vi "_fgv_range_tables.vi"(5 "Numeric Value in (0.0)":dbl, 6 "Range Tables (empty)":T2[](array[typedef]) {"Type" items=["Range", "Coerced", "Discrete"]}, 7 "Operation":T3=enum."Check", 8 "error in":errorcluster caption="error in (no error)", 9 "String value in (\"\")":string, 10 "Range Table ID in":string, 11 "VISA resource name":refnum<visa-resource-name>) -> (0 "error out":errorcluster, 1 "String Value out":string, 2 "Range Table Type out":T1, 3 "VISA resource name out":refnum<visa-resource-name>, 4 "Numeric Value out":dbl)   [LabVIEW 2020, in "Rohde&Schwarz RTx Oscilloscopes.lvlib" / "rsidr_core.lvlib"]
uses:
  rsidr_core.lvlib
  _type_Operation_Fgv_RangeTable.ctl
  type_Input_Format_RangeTable.ctl
  _type_RangeTable_Type.ctl
  type_Error_Codes.ctl
  type_AdditionalFlag_Bits.ctl
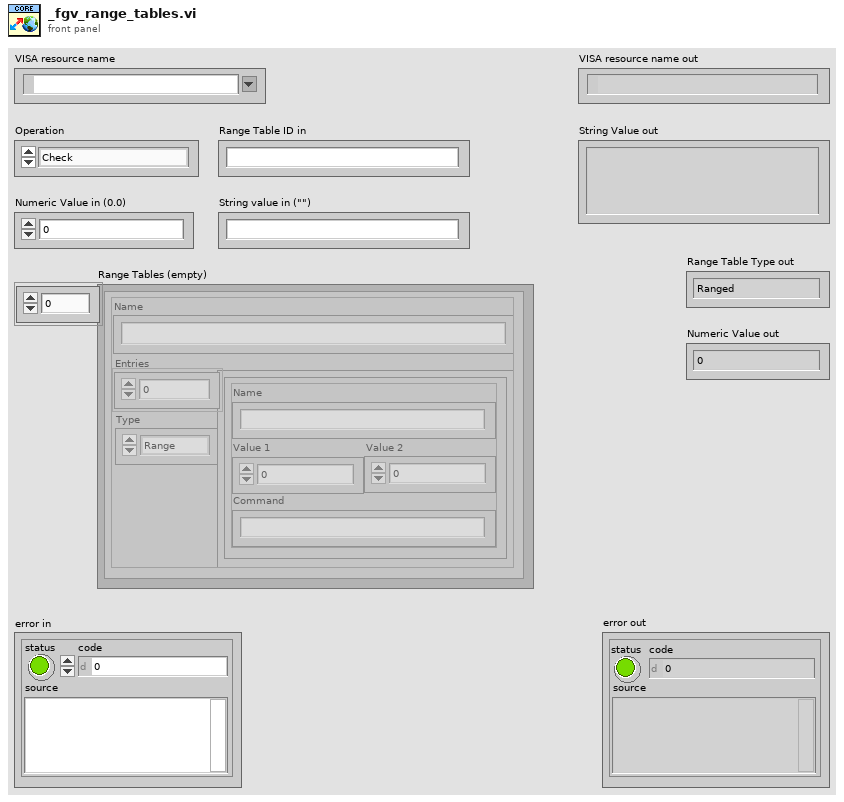
[diagram p1: front panel]
types:
  T1 = typedef "Rohde&Schwarz RTx Oscilloscopes.lvlib/rsidr_core.lvlib/_type_RangeTable_Type.ctl" = enum16{"Ranged", "Coerced", "Discrete"}
  T2 = typedef "Rohde&Schwarz RTx Oscilloscopes.lvlib/rsidr_core.lvlib/type_Input_Format_RangeTable.ctl" = cluster{"Type":u16, "Name":string, "Entries":cluster{"Name":string, "Value 1":dbl, "Value 2":dbl, "Command":string}[]}
  T3 = typedef "Rohde&Schwarz RTx Oscilloscopes.lvlib/rsidr_core.lvlib/_type_Operation_Fgv_RangeTable.ctl" = enum16{"Initialize", "Check", "Coerce", "Get Command String", "Get Numeric Value", "Get Default Value", "Get Range Table Type"}
  T4 = typedef "Rohde&Schwarz RTx Oscilloscopes.lvlib/rsidr_core.lvlib/type_Error_Codes.ctl" = enum16{"No_error", "VISA_err_ResourceNotFound", "VISA_err_Timeout", "VISA_warn_MoreDataAvailable", "RS_err_MissingCallback", "RS_err_InvalidAttribute", "RS_err_InvalidValue", "RS_err_UnknownResource", "RS_err_AlreadyInitialized", "RS_err_InstrumentStatus", "RS_err_BadRepCapName", "RS_err_TypesMismatch", "RS_err_ValueNotSupported", "RS_err_InvalidRngTable", "RS_err_IDqueryFail", "RS_err_UnexpResponse", "VISA_warn_ConfigNotLoaded", "RS_err_AttributeNotReadable", "RS_err_AttributeNotWritable", "RS_err_InstrumentType", "RS_err_InstrumentOption", "VISA_err_InvalidSize", "RS_err_ReliabilityIndicator", "VISA_warn_UnknownStatus", "VISA_warn_TermCharRead", "VISA_err_IO_error", "RS_err_FunctionNotSupported", "VISA_warn_QueueEmpty"}
  T5 = typedef "Rohde&Schwarz RTx Oscilloscopes.lvlib/rsidr_core.lvlib/type_AdditionalFlag_Bits.ctl" = enum16{"Send LF after Bin Block", "Junk read with io_clear_buffers.vi", "io_clear_buffers: viClear()", "io_clear_buffers: viFlush()", "<NotUsed1>", "Allow Dbl & Int Bin/Ascii read", "*OPC? in check_instrument_error.vi", "<NotUsed2>", "Smart Enum Matching", "Less Strict RepCaps check", "AssureResponseEndWithLF"}
  T6 = cluster{"Values":i32[], "FullCmd":string[], "ShortCmd":string[]}
  T7 = cluster{"Name":string, "Value 1":dbl, "Value 2":dbl, "Command":string}[]
  T8 = cluster{"Name":string, "Value 1":dbl, "Value 2":dbl, "Command":string}
  T9 = cluster{"Name":string, "Range Table Type":T1, "Variant":variant}
  T10 = cluster{"Name":string, "Range Table Type":T1, "Variant":variant}[]
  T11 = typedef "Rohde&Schwarz RTx Oscilloscopes.lvlib/rsidr_core.lvlib/type_Session_Data.ctl" = cluster{"IDN string":string, "Instrument FW":string, "Instr type":string, "Instr type for err. msg.":string, "Installed Options":string[], "Ignore Error Messages":string, "Logging params":variant, "OPC Timeout":i32, "VISA Timeout":i32, "STB Poll VISA Timeout":i32, "Additional Flags":i32, "Wait Before Read":i32, "Wait Before Write":i32, "Option String Flags":i32, "IO Segment Size":i64, "VISA Access Mode":T12, "Interface Type":T13, "OPC Wait Mode":T14, "Bin Float Number  Format":T15, "Bin Integer Number Format":T16, "Simulate":bool, "VXIcapable":bool, "Duplicate Session":bool, "Add LF to Write":bool, "Logging":bool, "Fast Sweep":bool, "Query Instrument Status":bool, "Check Range":bool, "Check Options":bool, "OPC-sync Attr Writes":bool, "OPC-sync Attr Queries":bool}
  T12 = typedef "Rohde&Schwarz RTx Oscilloscopes.lvlib/rsidr_core.lvlib/type_VisaAccessMode.ctl" = u16
  T13 = typedef "Rohde&Schwarz RTx Oscilloscopes.lvlib/rsidr_core.lvlib/type_InterfaceType.ctl" = enum16{"Unknown", "GPIB", "VXI", "GPIB_VXI", "ASRL", "PXI", "TCPIP", "USB", "SOCKET"}
  T14 = typedef "Rohde&Schwarz RTx Oscilloscopes.lvlib/rsidr_core.lvlib/type_OPC_Wait_Mode.ctl" = enum16{"STBpolling", "STBpollingSlow", "STBpollingSuperSlow", "ServiceRequest", "OPCquery"}
  T15 = typedef "Rohde&Schwarz RTx Oscilloscopes.lvlib/rsidr_core.lvlib/type_Binary_Float_Number_Format.ctl" = enum16{"Float_4_Bytes_Swapped", "Float_4_Bytes", "Double_8_Bytes_Swapped", "Double_8_Bytes"}
  T16 = typedef "Rohde&Schwarz RTx Oscilloscopes.lvlib/rsidr_core.lvlib/type_Binary_Integer_Number_Format.ctl" = enum16{"Int32_4_Bytes_Swapped", "Int32_4 Bytes", "Int16_2_Bytes_Swapped", "Int16_2_Bytes"}
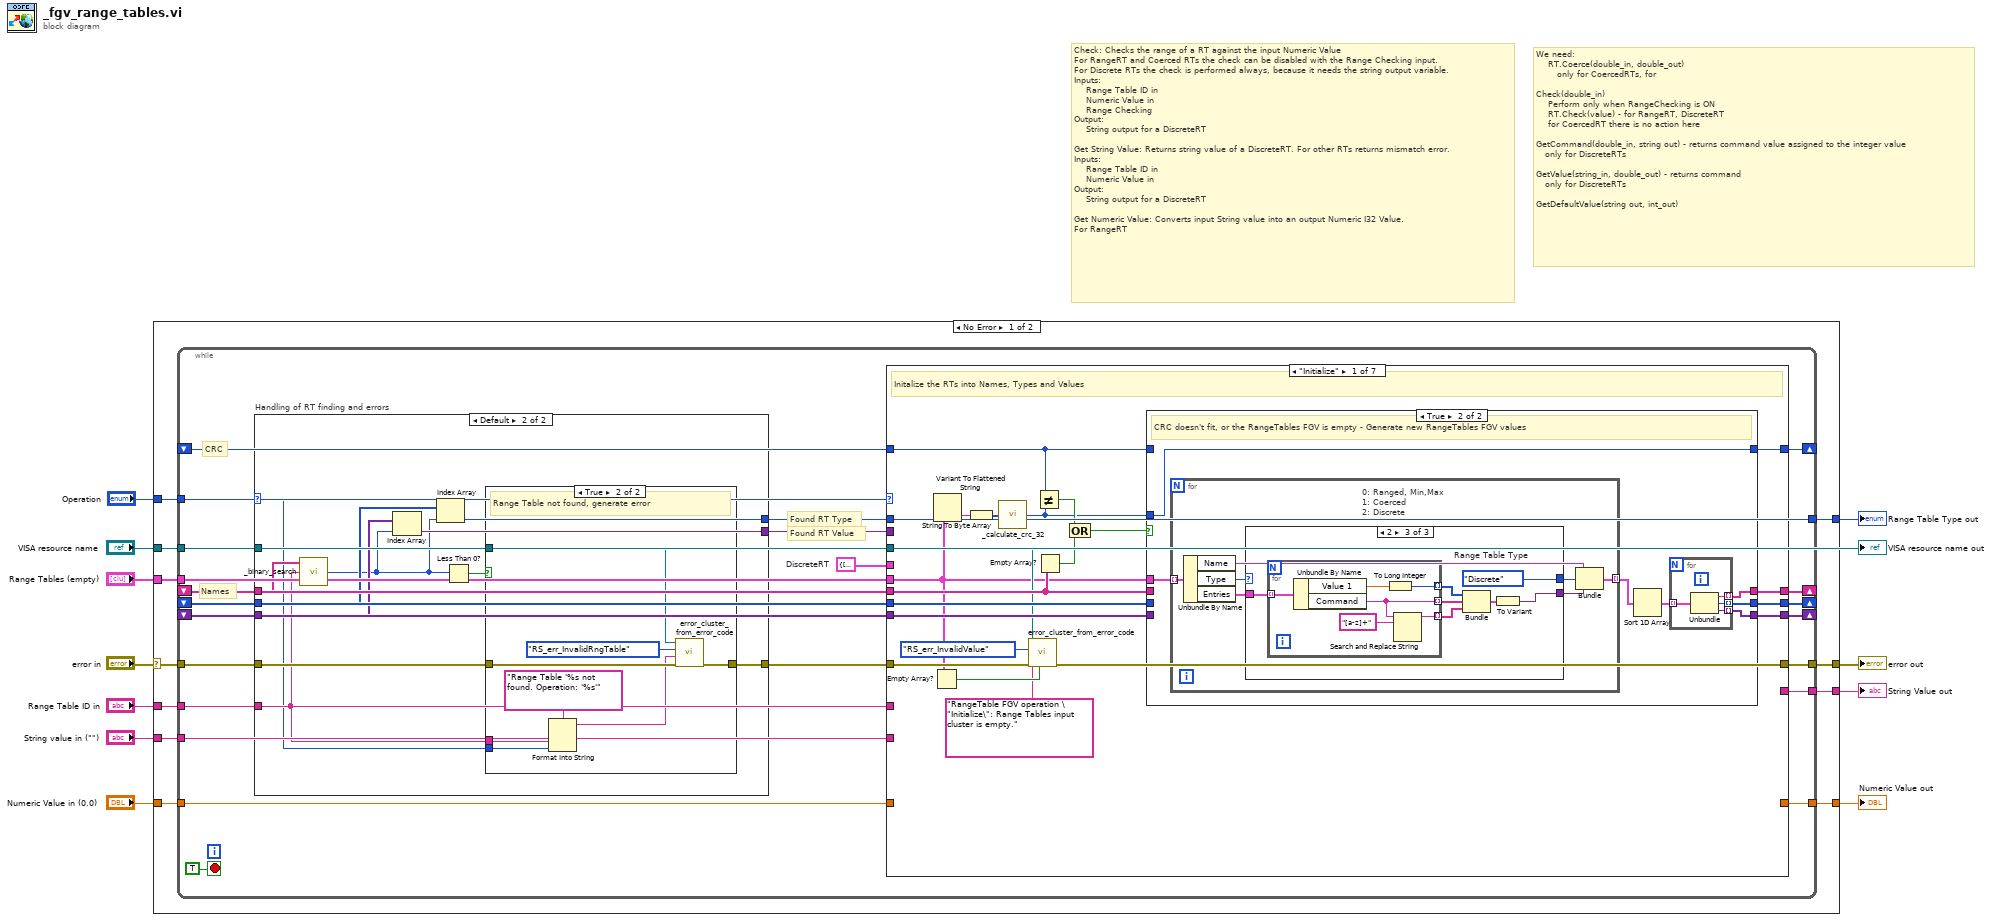
[diagram p0: block diagram]
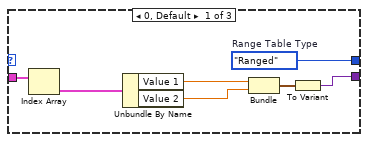
[diagram p5: hidden frame]
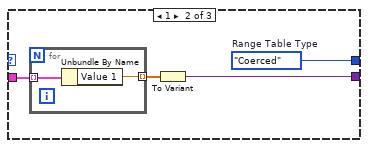
[diagram p6: hidden frame]
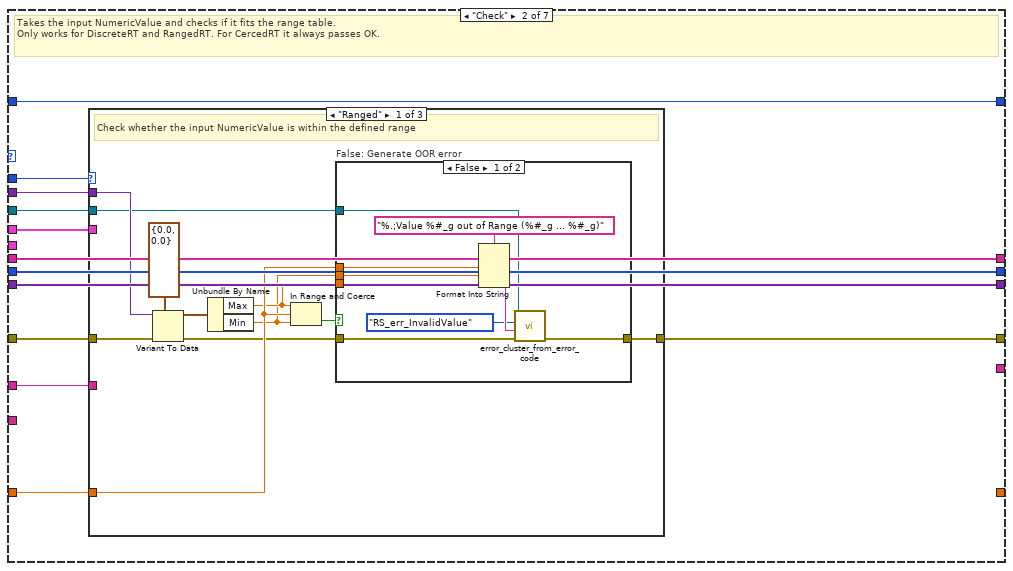
[diagram p7: hidden frame]
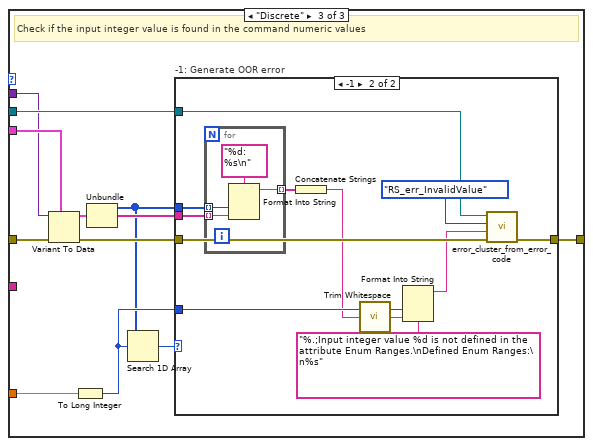
[diagram p10: hidden frame]
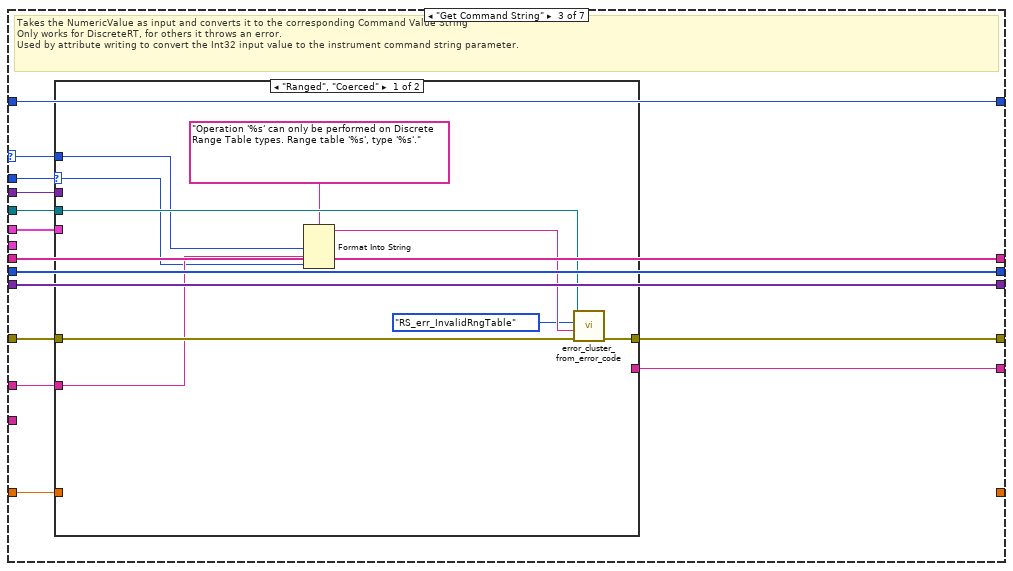
[diagram p12: hidden frame]
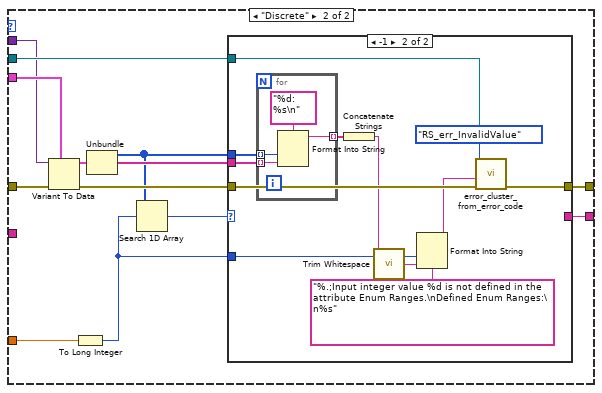
[diagram p13: hidden frame]
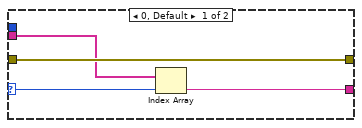
[diagram p14: hidden frame]
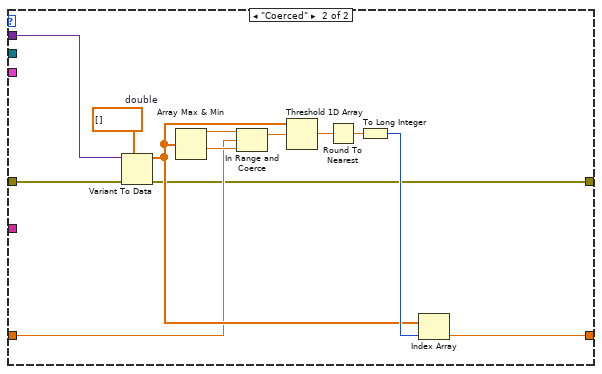
[diagram p16: hidden frame]
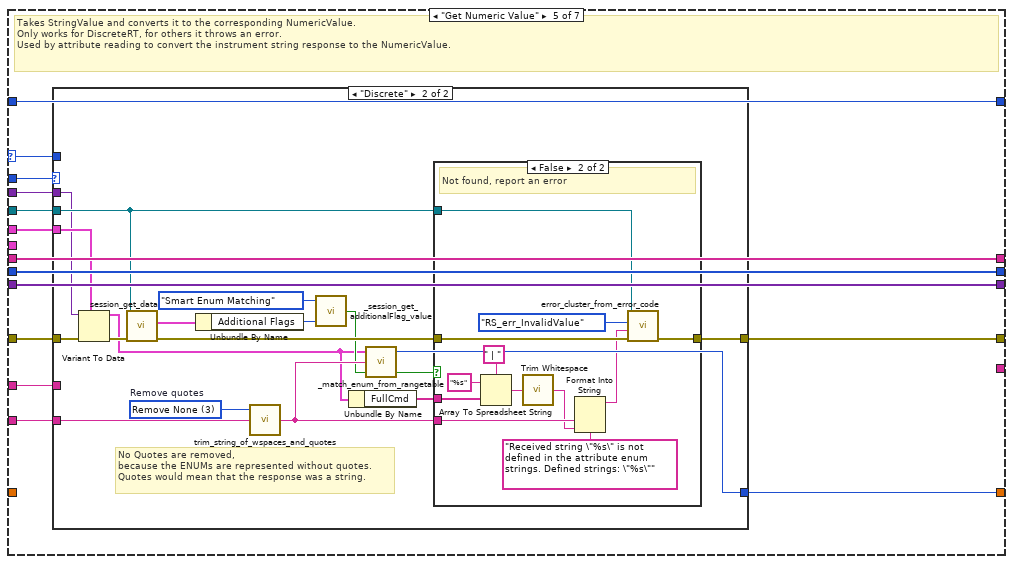
[diagram p17: hidden frame]
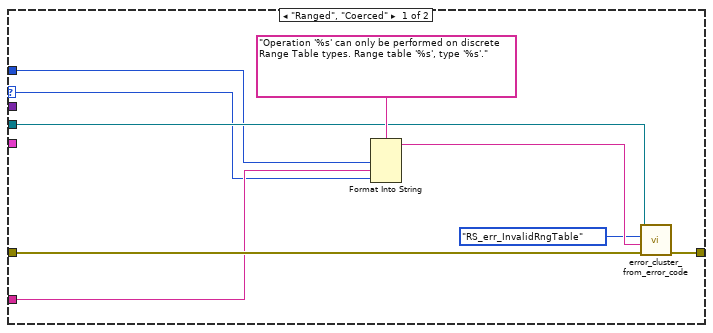
[diagram p18: hidden frame]
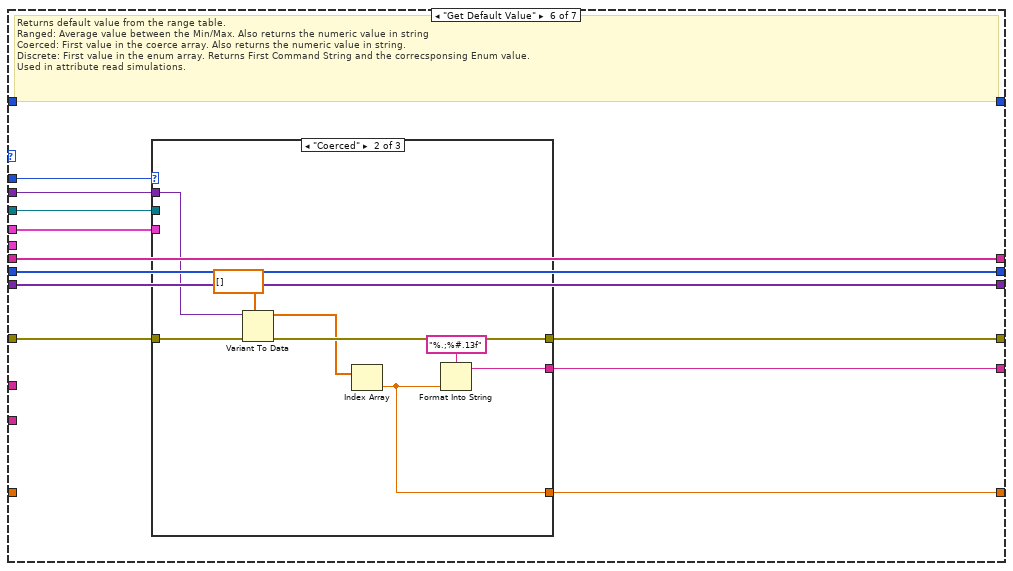
[diagram p20: hidden frame]
diagram:
  # "We need:\n    RT.Coerce(double_in, double_out)\n       only for CoercedRTs, for \n\nCheck(double_in)\n    Perform only when RangeChecking is ON\n    RT.Check(value) - for RangeRT, DiscreteRT\n    for CoercedRT there is no action here\n\nGetCommand(double_in, string out) - returns command value assigned to the integer value\n   only for DiscreteRTs\n\nGetValue(string_in, double_out) - returns command \n   only for DiscreteRTs\n\nGetDefaultValue(string out, int_out)"
  # "Check: Checks the range of a RT against the input Numeric Value\nFor RangeRT and Coerced RTs the check can be disabled with the Range Checking input.\nFor Discrete RTs the check is performed always, because it needs the string output variable.\nInputs:\n    Range Table ID in\n    Numeric Value in\n    Range Checking\nOutput:\n    String output for a DiscreteRT\n\nGet String Value: Returns string value of a DiscreteRT. For other RTs returns mismatch error.\nInputs:\n    Range Table ID in\n    Numeric Value in\nOutput:\n    String output for a DiscreteRT\n\nGet Numeric Value: Converts input String value into an output Numeric I32 Value.\nFor RangeRT"
  n1 = case shown="No Error" "error in" {
    selector: "error in" -> [w18 w384]
    tunnel: "Operation" -> [w22 _]
    tunnel: [w17 w384] -> w7
    tunnel: "Range Table ID in" -> [w21 _]
    tunnel: "Numeric Value in (0.0)" -> [w20 w383]
    tunnel: "String value in (\"\")" -> [w19 _]
    tunnel: [w16 _] -> w6
    tunnel: "VISA resource name" -> [w15 _]
    tunnel: "Range Tables (empty)" -> [w14 _]
    tunnel: [w13 w383] -> w2
    tunnel: [w12 _] -> w1
    frame No Error {
      n2 = while {
        tunnel: w22 -> [w32]
        tunnel: w21 -> [w34]
        tunnel: w20 -> [w45]
        tunnel: w19 -> [w44]
        tunnel: w18 -> [w31]
        tunnel: [w43] -> w17
        tunnel: [w42] -> w16
        shift-right: [w41] -> _
        shift-left: _ -> [w29]
        shift-right: [w39] -> _
        shift-left: _ -> [w27]
        shift-right: [w38] -> _
        shift-left: _ -> [w33]
        shift-right: [w36] -> _
        shift-left: _ -> [w37]
        tunnel: w15 -> [w28]
        tunnel: w14 -> [w35]
        tunnel: [w24] -> w13
        tunnel: [w23] -> w12
        stop <- TRUE stop-if-true
        w25 = T6 {"Values"=[], "FullCmd"=[], "ShortCmd"=[]}  # DiscreteRT
        # "Found RT Value"
        # "Found RT Type"
        # "CRC"
        # "Names"
        n3 = case "Handling of RT finding and errors" shown="Default" w32 {
          selector: w32 -> [_ w49]
          tunnel: w34 -> [_ w53]
          tunnel: w33 -> [_ w55]
          tunnel: w31 -> [w46 w57]
          tunnel: [w46 w58] -> w30
          tunnel: w29 -> [_ w54]
          tunnel: w28 -> [_ w56]
          tunnel: w27 -> [_ w52]
          tunnel: [_ w51] -> w26
          tunnel: [_ w50] -> w23
          frame "Initialize" {
          }
          frame Default {
            n4 = call "_binary_search.vi"("String to search"=w53, "Strings in"=w55) -> ("Index out"=w48:i32)  [unwired: 3 in]
            n5 = Index Array(array=w52, index=w48) -> (element=w51:variant)
            n6 = Index Array(array=w54, index=w48) -> (element=w50:T1)
            n7 = Less Than 0?(x=w48) -> (x < 0?=w47:bool)
            n8 = case shown="True" w47 {
              tunnel: [w59 w66] -> w58
              tunnel: w57 -> [w59 w65]
              tunnel: w56 -> [_ w64]
              tunnel: w53 -> [_ w63]
              tunnel: w49 -> [_ w60]
              frame False {
              }
              frame True {
                # "Range Table not found, generate error"
                n9 = Format Into String(format string="Range Table '%s not found. Operation: '%s'" ("string"), w63, w60) -> (resulting string=w62:string)  [unwired: 2 in, 1 out]
                n10 = call "error_cluster_from_error_code.vi"("error in"=w65, "Error Message (\"\")"=w62, "Error Enum in"=type_Error_Codes."RS_err_InvalidRngTable", "VISA resource name"=w64) -> ("error out"=w66:errorcluster)  [unwired: 6 in, 1 out]
              }
            }
          }
        }
        n11 = case shown="\"Initialize\"" w32 {
          selector: w32 -> [_ _ w200 w257 w286 _ _]
          tunnel: [w86 w148 w213 w269 w298 w349 w378] -> w43
          tunnel: w34 -> [_ w140 w204 w261 w295 _ _]
          tunnel: w44 -> [_ _ _ _ w297 _ _]
          tunnel: w45 -> [_ w147 w212 w268 _ _ _]
          tunnel: w30 -> [w85 w145 w209 w266 w294 w347 w378]
          tunnel: [_ _ w211 _ _ w342 _] -> w42
          tunnel: w29 -> [w80 w143 w207 w264 w293 w345 w379]
          tunnel: [w88 w143 w207 w264 w293 w345 w379] -> w41
          tunnel: w27 -> [w79 w144 w208 w265 w292 w346 w381]
          tunnel: [w87 w144 w208 w265 w292 w346 w381] -> w39
          tunnel: [w84 w146 w210 w267 w296 w348 w382] -> w38
          tunnel: w33 -> [w77 w146 w210 w267 w296 w348 w382]
          tunnel: w37 -> [w74 w142 w206 w263 w291 w344 w380]
          tunnel: [w73 w142 w206 w263 w291 w344 w380] -> w36
          tunnel: w28 -> [w69 w141 w205 w262 w290 w343 _]
          tunnel: w35 -> [w68 _ _ _ _ _ _]
          tunnel: w25 -> [_ w139 w203 w260 w289 w341 _]
          tunnel: w23 -> [_ w138 w201 w258 w287 w340 _]
          tunnel: w26 -> [_ w137 w202 w259 w288 w339 _]
          tunnel: [_ _ _ w256 w285 w338 _] -> w24
          frame "Initialize" {
            # "Initalize the RTs into Names, Types and Values"
            n12 = Empty Array?(array=w68) -> (empty?=w78:bool)
            n13 = Variant To Flattened String(Variant=w68) -> (data string=w83:string)  [unwired: 1 out]
            n14 = String To Byte Array(string=w83) -> (unsigned byte array=w82:u8[])
            n15 = call "_calculate_crc_32.vi"("Data in"=w82) -> ("CRC_32"=w72:u32)  [unwired: 4 in]
            n16 = call "error_cluster_from_error_code.vi"("Error Creation Enabled (True)"=w78, "error in"=w85, "Error Message (\"\")"="RangeTable FGV operation \"Initialize\": Range Tables input cluster is empty." ("format string"), "Error Enum in"=type_Error_Codes."RS_err_InvalidValue", "VISA resource name"=w69) -> ("error out"=w86:errorcluster)  [unwired: 5 in, 1 out]
            n17 = Not Equal?(x=w74, y=w72) -> (x != y?=w76:bool)
            n18 = Empty Array?(array=w77) -> (empty?=w75:bool)
            n19 = Compound Arithmetic op=OR(w76, w75) -> (w81:bool)
            n20 = case shown="True" w81 {
              tunnel: [w91 w98] -> w88
              tunnel: [w90 w97] -> w87
              tunnel: w68 -> [_ w95]
              tunnel: [w92 w94] -> w84
              tunnel: w77 -> [w92 _]
              tunnel: w80 -> [w91 _]
              tunnel: w79 -> [w90 _]
              tunnel: w74 -> [w89 _]
              tunnel: [w89 w93] -> w73
              tunnel: w72 -> [_ w93]
              frame False {
              }
              frame True {
                # "CRC doesn't fit, or the RangeTables FGV is empty - Generate new RangeTables FGV values"
                n21 = for {
                  tunnel: w95 -> [w110] mode=indexing
                  tunnel: [w105] -> w99 mode=indexing
                  n22 = Unbundle By Name(w110) -> ("Name"=w108:string, "Type"=w107:u16, "Entries"=w109:T7)
                  n23 = case "0: Ranged, Min,Max\n1: Coerced\n2: Discrete" shown="2" w107 {
                    tunnel: w109 -> [w117 w121 w130]
                    tunnel: [w112 w119 w129] -> w106
                    tunnel: [w111 w118 w124] -> w104
                    frame 0, Default {
                      w111 = _type_RangeTable_Type."Ranged"  # Range Table Type
                      n24 = Index Array(array=w117) -> (element=w116:T8)  [unwired: 1 in]
                      n25 = Unbundle By Name(w116) -> ("Value 1"=w114:dbl, "Value 2"=w115:dbl)
                      n26 = Bundle("Value 1"=w114, "Value 2"=w115) -> (w113:cluster{"Value 1":dbl, "Value 2":dbl})  [unwired: 1 in]
                      n27 = To Variant(anything=w113) -> (Variant=w112:variant)
                    }
                    frame 1 {
                      w118 = _type_RangeTable_Type."Coerced"  # Range Table Type
                      n28 = for {
                        tunnel: [w123] -> w120 mode=indexing
                        tunnel: w121 -> [w122] mode=indexing
                        n29 = Unbundle By Name(w122) -> ("Value 1"=w123:dbl)
                      }
                      n30 = To Variant(anything=w120) -> (Variant=w119:variant)
                    }
                    frame 2 {
                      w124 = _type_RangeTable_Type."Discrete"  # Range Table Type
                      n31 = for {
                        tunnel: w130 -> [w136] mode=indexing
                        tunnel: [w132] -> w127 mode=indexing
                        tunnel: [w134] -> w126 mode=indexing
                        tunnel: [w131] -> w125 mode=indexing
                        n32 = Unbundle By Name(w136) -> ("Value 1"=w135:dbl, "Command"=w132:string)
                        n33 = To Long Integer(number=w135) -> (32bit integer=w134:i32)
                        n34 = Search and Replace String(input string=w132, search string="[a-z]+") -> (result string=w131:string)  [unwired: 6 in, 3 out]
                      }
                      n35 = Bundle(w126, w127, w125) -> (w128:cluster{i32[], string[], string[]})  [unwired: 1 in]
                      n36 = To Variant(anything=w128) -> (Variant=w129:variant)
                    }
                  }
                  n37 = Bundle("Name"=w108, "Range Table Type"=w104, "Variant"=w106) -> (w105:T9)  [unwired: 1 in]
                }
                n38 = Sort 1D Array(array=w99) -> (sorted array=w96:T10)
                n39 = for {
                  tunnel: w96 -> [w102] mode=indexing
                  tunnel: [w103] -> w94 mode=indexing
                  tunnel: [w101] -> w98 mode=indexing
                  tunnel: [w100] -> w97 mode=indexing
                  n40 = Unbundle(w102) -> ("Name"=w103:string, "Range Table Type"=w101:T1, "Variant"=w100:variant)
                }
              }
            }
          }
          frame "Check" {
            # "Takes the input NumericValue and checks if it fits the range table.\nOnly works for DiscreteRT and RangedRT. For CercedRT it always passes OK."
            n41 = case shown="\"Ranged\"" w138 {
              tunnel: w147 -> [w158 _ w175]
              tunnel: [w159 w170 w179] -> w148
              tunnel: w145 -> [w157 w170 w182]
              tunnel: w140 -> [_ _ _]
              tunnel: w141 -> [w152 _ w173]
              tunnel: w139 -> [_ _ w172]
              tunnel: w137 -> [w153 _ w171]
              frame "Ranged" {
                # "Check whether the input NumericValue is within the defined range"
                n42 = Variant To Data(error in=w157, type=cluster{"Min":dbl, "Max":dbl} {"Min"=0.0, "Max"=0.0} ("output cluster"), Variant=w153) -> (data=w151:cluster{"Min":dbl, "Max":dbl}, error out=w154:errorcluster)
                n43 = Unbundle By Name(w151) -> ("Max"=w150:dbl, "Min"=w149:dbl)
                n44 = In Range and Coerce(upper limit=w150, x=w158, lower limit=w149) -> (In Range?=w156:bool)  [unwired: 1 out]
                n45 = case "False: Generate OOR error" shown="False" w156 {
                  tunnel: w158 -> [w167 _]
                  tunnel: w154 -> [w166 w169]
                  tunnel: [w165 w169] -> w159
                  tunnel: w149 -> [w164 _]
                  tunnel: w150 -> [w163 _]
                  tunnel: w152 -> [w160 _]
                  frame False {
                    n46 = Format Into String(format string="%.;Value %#_g out of Range (%#_g ... %#_g)" ("string"), w167, w164, w163) -> (resulting string=w162:string)  [unwired: 2 in, 1 out]
                    n47 = call "error_cluster_from_error_code.vi"("error in"=w166, "Error Message (\"\")"=w162, "Error Enum in"=type_Error_Codes."RS_err_InvalidValue", "VISA resource name"=w160) -> ("error out"=w165:errorcluster)  [unwired: 6 in, 1 out]
                  }
                  frame True {
                  }
                }
              }
              frame "Coerced" {
                # "CoercedRT value check is always PASS"
              }
              frame "Discrete" {
                # "Check if the input integer value is found in the command numeric values"
                n48 = Variant To Data(error in=w182, type=w172, Variant=w171) -> (data=w181:T6, error out=w180:errorcluster)
                n49 = To Long Integer(number=w175) -> (32bit integer=w177:i32)
                n50 = Unbundle(w181) -> ("Values"=w174:i32[], "FullCmd"=w176:string[])  [unwired: 1 out]
                n51 = Search 1D Array(1D array=w174, element=w177) -> (index of element=w178:i32)  [unwired: 1 in]
                n52 = case "-1: Generate OOR error" shown="-1" w178 {
                  tunnel: w177 -> [_ w194]
                  tunnel: w180 -> [w183 w193]
                  tunnel: [w183 w192] -> w179
                  tunnel: w176 -> [_ w190]
                  tunnel: w174 -> [_ w191]
                  tunnel: w173 -> [_ w186]
                  frame Default {
                  }
                  frame -1 {
                    n53 = for {
                      tunnel: w191 -> [w199] mode=indexing
                      tunnel: w190 -> [w198] mode=indexing
                      tunnel: [w196] -> w189 mode=indexing
                      n54 = Format Into String(format string="%d: %s\n", w199, w198) -> (resulting string=w196:string)  [unwired: 2 in, 1 out]
                    }
                    n55 = Concatenate Strings(w189) -> (w185:string)
                    n56 = call "Trim Whitespace.vi"("string"=w185) -> ("trimmed string"=w188:string)  [unwired: 1 in]
                    n57 = Format Into String(format string="%.;Input integer value %d is not defined in the attribute Enum Ranges.\nDefined Enum Ranges:\n%s" ("string"), w194, w188) -> (resulting string=w187:string)  [unwired: 2 in, 1 out]
                    n58 = call "error_cluster_from_error_code.vi"("error in"=w193, "Error Message (\"\")"=w187, "Error Enum in"=type_Error_Codes."RS_err_InvalidValue", "VISA resource name"=w186) -> ("error out"=w192:errorcluster)  [unwired: 6 in, 1 out]
                  }
                }
              }
            }
          }
          frame "Get Command String" {
            # "Takes the NumericValue as input and converts it to the corresponding Command Value String\nOnly works for DiscreteRT, for others it throws an error.\nUsed by attribute writing to convert the Int32 input value to the instrument command string parameter."
            n59 = case shown="\"Ranged\", \"Coerced\"" w201 {
              selector: w201 -> [w215 _]
              tunnel: w212 -> [_ w227]
              tunnel: [w221 w232] -> w213
              tunnel: w209 -> [w222 w235]
              tunnel: [_ w228] -> w211
              tunnel: w204 -> [w220 _]
              tunnel: w205 -> [w217 w225]
              tunnel: w203 -> [_ w224]
              tunnel: w202 -> [_ w223]
              tunnel: w200 -> [w214 _]
              frame "Ranged", "Coerced" {
                n60 = Format Into String(format string="Operation '%s' can only be performed on Discrete Range Table types. Range table '%s', type '%s'." ("string"), w214, w220, w215) -> (resulting string=w219:string)  [unwired: 2 in, 1 out]
                n61 = call "error_cluster_from_error_code.vi"("error in"=w222, "Error Message (\"\")"=w219, "Error Enum in"=type_Error_Codes."RS_err_InvalidRngTable", "VISA resource name"=w217) -> ("error out"=w221:errorcluster)  [unwired: 6 in, 1 out]
              }
              frame "Discrete" {
                n62 = Variant To Data(error in=w235, type=w224, Variant=w223) -> (data=w234:T6, error out=w233:errorcluster)
                n63 = To Long Integer(number=w227) -> (32bit integer=w230:i32)
                n64 = Unbundle(w234) -> ("Values"=w226:i32[], "FullCmd"=w229:string[])  [unwired: 1 out]
                n65 = Search 1D Array(1D array=w226, element=w230) -> (index of element=w231:i32)  [unwired: 1 in]
                n66 = case shown="-1" w231 {
                  selector: w231 -> [w238 _]
                  tunnel: w230 -> [_ w250]
                  tunnel: w233 -> [w239 w249]
                  tunnel: [w239 w248] -> w232
                  tunnel: w229 -> [w237 w246]
                  tunnel: [w236 _] -> w228
                  tunnel: w226 -> [_ w247]
                  tunnel: w225 -> [_ w240]
                  frame 0, Default {
                    n67 = Index Array(array=w237, index=w238) -> (element=w236:string)
                  }
                  frame -1 {
                    n68 = for {
                      tunnel: w247 -> [w255] mode=indexing
                      tunnel: w246 -> [w254] mode=indexing
                      tunnel: [w252] -> w245 mode=indexing
                      n69 = Format Into String(format string="%d: %s\n", w255, w254) -> (resulting string=w252:string)  [unwired: 2 in, 1 out]
                    }
                    n70 = Concatenate Strings(w245) -> (w244:string)
                    n71 = call "Trim Whitespace.vi"("string"=w244) -> ("trimmed string"=w243:string)  [unwired: 1 in]
                    n72 = Format Into String(format string="%.;Input integer value %d is not defined in the attribute Enum Ranges.\nDefined Enum Ranges:\n%s" ("string"), w250, w243) -> (resulting string=w242:string)  [unwired: 2 in, 1 out]
                    n73 = call "error_cluster_from_error_code.vi"("error in"=w249, "Error Message (\"\")"=w242, "Error Enum in"=type_Error_Codes."RS_err_InvalidValue", "VISA resource name"=w240) -> ("error out"=w248:errorcluster)  [unwired: 6 in, 1 out]
                  }
                }
              }
            }
          }
          frame "Coerce" {
            # "Takes the input NumericValue as input and coerces it to the nearest value in the Range Table. The value comes out in the Numeric Double Value out.\nOnly performs a coersion for the CoerceRT, for others it returns the input value.\nUsed by attribute writing to coerce the values before writing to the instrument."
            n74 = case shown="\"Ranged\", \"Discrete\"" w258 {
              tunnel: w268 -> [w271 w274]
              tunnel: [w270 w272] -> w269
              tunnel: w266 -> [w270 w276]
              tunnel: w261 -> [_ _]
              tunnel: w262 -> [_ _]
              tunnel: w260 -> [_ _]
              tunnel: w259 -> [_ w275]
              tunnel: w257 -> [_ _]
              tunnel: [w271 w273] -> w256
              frame "Ranged", "Discrete" {
              }
              frame "Coerced" {
                w284 = dbl[] []  # double
                n75 = Variant To Data(error in=w276, type=w284, Variant=w275) -> (data=w277:dbl[], error out=w272:errorcluster)
                n76 = Array Max & Min(array=w277) -> (max value=w283:dbl, min value=w282:dbl)  [unwired: 2 out]
                n77 = In Range and Coerce(upper limit=w283, x=w274, lower limit=w282) -> (coerced(x)=w281:dbl)  [unwired: 1 out]
                n78 = Threshold 1D Array(2:w281, 3:w277) -> (0:w280:dbl)  [unwired: 1 in]
                n79 = Round To Nearest(number=w280) -> (nearest integer value=w279:dbl)
                n80 = To Long Integer(number=w279) -> (32bit integer=w278:i32)
                n81 = Index Array(array=w277, index=w278) -> (element=w273:dbl)
              }
            }
          }
          frame "Get Numeric Value" {
            # "Takes StringValue and converts it to the corresponding NumericValue.\nOnly works for DiscreteRT, for others it throws an error.\nUsed by attribute reading to convert the instrument string response to the NumericValue."
            n82 = case shown="\"Discrete\"" w287 {
              selector: w287 -> [w299 _]
              tunnel: [w304 w325] -> w298
              tunnel: [_ w310] -> w285
              tunnel: w297 -> [_ w319]
              tunnel: w294 -> [w303 w324]
              tunnel: w295 -> [w300 _]
              tunnel: w290 -> [w302 w322]
              tunnel: w289 -> [_ w317]
              tunnel: w288 -> [_ w308]
              tunnel: w286 -> [w301 _]
              frame "Ranged", "Coerced" {
                n83 = Format Into String(format string="Operation '%s' can only be performed on discrete Range Table types. Range table '%s', type '%s'." ("string"), w301, w300, w299) -> (resulting string=w307:string)  [unwired: 2 in, 1 out]
                n84 = call "error_cluster_from_error_code.vi"("error in"=w303, "Error Message (\"\")"=w307, "Error Enum in"=type_Error_Codes."RS_err_InvalidRngTable", "VISA resource name"=w302) -> ("error out"=w304:errorcluster)  [unwired: 6 in, 1 out]
              }
              frame "Discrete" {
                w318 = u16 3 items=["Remove All Quotes", "Remove Single Quotes", "Remove Double Quotes", "Remove None"]  # Remove quotes
                # "No Quotes are removed,\nbecause the ENUMs are represented without quotes.\nQuotes would mean that the response was a string."
                n85 = Variant To Data(error in=w324, type=w317, Variant=w308) -> (data=w312:T6, error out=w323:errorcluster)
                n86 = call "session_get_data.vi"("error in"=w323, "VISA resource name"=w322) -> ("error out"=w320:errorcluster, "Session User Data out"=w321:T11)  [unwired: 6 in, 2 out]
                n87 = Unbundle By Name(w321) -> ("Additional Flags"=w316:i32)
                n88 = call "trim_string_of_wspaces_and_quotes.vi"("String in"=w319, "Remove quotes (Remove All)"=w318) -> ("String out"=w315:string)  [unwired: 3 in]
                n89 = call "_session_get_additionalFlag_value.vi"("AdditionalFlags value in"=w316, "AdditionalFlag bit"=type_AdditionalFlag_Bits."Smart Enum Matching") -> ("AdditionalFlag bit value out"=w314:bool)  [unwired: 3 in]
                n90 = Unbundle By Name(w312) -> ("FullCmd"=w311:string[])
                n91 = call "_match_enum_from_rangetable.vi"("Smart matching"=w314, "Enum string to match"=w315, "Enums in"=w312) -> ("Success"=w313:bool, "Enum Value out"=w310:i32)  [unwired: 1 in]
                n92 = case shown="False" w313 {
                  tunnel: [_ w337] -> w325
                  tunnel: w320 -> [_ w335]
                  tunnel: w315 -> [_ w336]
                  tunnel: w311 -> [_ w334]
                  tunnel: w322 -> [_ w327]
                  frame True {
                    # "Success"
                  }
                  frame False {
                    # "Not found, report an error"
                    n93 = Array To Spreadsheet String(delimiter (Tab)=" | ", array=w334, 3:"%s" ("format string")) -> (spreadsheet string=w330:string)
                    n94 = call "Trim Whitespace.vi"("string"=w330) -> ("trimmed string"=w329:string)  [unwired: 1 in]
                    n95 = Format Into String(format string="Received string \"%s\" is not defined in the attribute enum strings. Defined strings: \"%s\"", w336, w329) -> (resulting string=w326:string)  [unwired: 2 in, 1 out]
                    n96 = call "error_cluster_from_error_code.vi"("error in"=w335, "Error Message (\"\")"=w326, "Error Enum in"=type_Error_Codes."RS_err_InvalidValue", "VISA resource name"=w327) -> ("error out"=w337:errorcluster)  [unwired: 6 in, 1 out]
                  }
                }
              }
            }
          }
          frame "Get Default Value" {
            # "Returns default value from the range table.\nRanged: Average value between the Min/Max. Also returns the numeric value in string\nCoerced: First value in the coerce array. Also returns the numeric value in string.\nDiscrete: First value in the enum array. Returns First Command String and the correcsponsing Enum value.\nUsed in attribute read simulations."
            n97 = case shown="\"Coerced\"" w340 {
              tunnel: [w354 w366 w375] -> w349
              tunnel: w347 -> [w360 w368 w377]
              tunnel: w343 -> [_ _ _]
              tunnel: [w352 w363 w373] -> w342
              tunnel: w341 -> [_ _ w372]
              tunnel: w339 -> [w351 w362 w371]
              tunnel: [w350 w361 w369] -> w338
              frame "Ranged" {
                n98 = Variant To Data(error in=w360, type=cluster{"Min":dbl, "Max":dbl} {"Min"=0.0, "Max"=0.0} ("output cluster"), Variant=w351) -> (data=w358:cluster{"Min":dbl, "Max":dbl}, error out=w354:errorcluster)
                n99 = Unbundle(w358) -> ("Min"=w357:dbl, "Max"=w356:dbl)
                n100 = Add(x=w357, y=w356) -> (x+y=w355:dbl)
                n101 = expression code="x/2"(w355) -> (w350:dbl)
                n102 = Format Into String(format string="%.;%#.13f", w350) -> (resulting string=w352:string)  [unwired: 2 in, 1 out]
              }
              frame "Coerced" {
                n103 = Variant To Data(error in=w368, type=dbl[] [], Variant=w362) -> (data=w365:dbl[], error out=w366:errorcluster)
                n104 = Index Array(array=w365) -> (element=w361:dbl)  [unwired: 1 in]
                n105 = Format Into String(format string="%.;%#.13f", w361) -> (resulting string=w363:string)  [unwired: 2 in, 1 out]
              }
              frame "Discrete" {
                n106 = Variant To Data(error in=w377, type=w372, Variant=w371) -> (data=w376:T6, error out=w375:errorcluster)
                n107 = Unbundle(w376) -> ("Values"=w370:i32[], "FullCmd"=w374:string[])  [unwired: 1 out]
                n108 = Index Array(array=w374) -> (element=w373:string)  [unwired: 1 in]
                n109 = Index Array(array=w370) -> (element=w369:i32)  [unwired: 1 in]
              }
            }
          }
          frame "Get Range Table Type" {
          }
        }
      }
    }
    frame Error {
    }
  }
  "error out" <- w7
  "String Value out" <- w6
  "Numeric Value out" <- w2
  "Range Table Type out" <- w1
  "VISA resource name out" <- "VISA resource name"
